vi "EmptyString.vi"() -> ()   [LabVIEW 2019]
panel:
  in  "Hardware":string
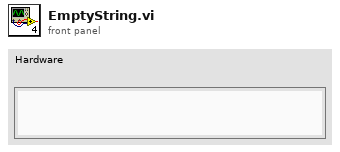
[diagram p1: front panel]
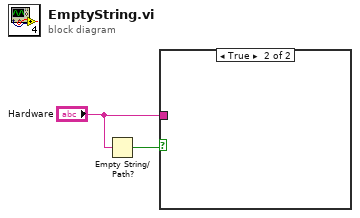
[diagram p0: block diagram]
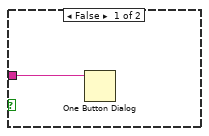
[diagram p2: hidden frame]
diagram:
  n1 = Empty String/Path?(string/path="Hardware") -> (empty?=w2:bool)
  n2 = case shown="True" w2 {
    tunnel: "Hardware" -> [w3 _]
    frame False {
      n3 = One Button Dialog(message=w3) -> ()  [unwired: 1 in, 1 out]
    }
    frame True {
    }
  }
